vi "Camera setup.vi"() -> ()   [LabVIEW 2012]
uses:
  <vilib>/userDefined/High Color/IMAQdx.ctl
  <vilib>/vision/Calibration.llb/Calibration Reference Points.ctl
  <vilib>/vision/driver/NI_Vision_Acquisition_Software.lvlib
  <vilib>/vision/NI_Vision_Development_Module.lvlib
panel:
  out "ROI":T1
  in  "Attributes":string="[NIIMAQ_HEADER]\nType = 2\nVersion = 8\n\n[CAMERA_DATA]\nAcquisitionAttributes::Bayer::GainB = \"1\"\nAcquisitionAttributes::Bayer::GainG = \"1\"\nAcquisitionAttributes::Bayer::GainR = \"1\"\nAcquisitionAttributes::Bayer::Pattern = \"Use hardware value\"\nAcquisitionAttributes::BitsPerPixel = \"Use hardware value\"\nAcquisitionAttributes::IgnoreFirstFrame = \"false\"\nAcquisitionAttributes::OverwriteMode = \"Get Newest\"\nAcquisitionAttributes::PixelSignedness = \"Signed\"\nAcquisitionAttributes::ReceiveTimestampMode = \"None\"\nAcquisitionAttributes::ShiftPixelBits = \"false\"\nAcquisitionAttributes::SwapPixelBytes = \"false\"\nAcquisitionAttributes::Timeout = \"5000\"\nAcquisitionAttributes::VerticalMirror = \"false\"\nAcquisitionAttributes::VideoMode = \"960x720 RGB24 15.00fps\"\nCameraAttributes::BacklightCompensation::Mode = \"Manual\"\nCameraAttributes::BacklightCompensation::Value = \"false\"\nCameraAttributes::Brightness::Mode = \"Manual\"\nCameraAttributes::Brightness::Value = \"128\"\nCameraAttributes::Contrast::Mode = \"Manual\"\nCameraAttributes::Contrast::Value = \"0.27000000000000002\"\nCameraAttributes::Exposure::Mode = \"Manual\"\nCameraAttributes::Exposure::Value = \"0.015625\"\nCameraAttributes::Gain::Mode = \"Manual\"\nCameraAttributes::Gain::Value = \"254\"\nCameraAttributes::Saturation::Mode = \"Manual\"\nCameraAttributes::Saturation::Value = \"28\"\nCameraAttributes::Sharpness::Mode = \"Manual\"\nCameraAttributes::Sharpness::Value = \"180\"\nCameraAttributes::WhiteBalance::Mode = \"Manual\"\nCameraAttributes::WhiteBalance::Value = \"6299\"\n"
  out "Tank":dbl(slide) scale=0.0..300.0
  in  "Stop Acquisition":bool
  in  "millisecond multiple":u32
  in  "Continuous Acquire image":bool
  out "min index":i32
  out "Gray":T2(plugin-control)
  in  "Smooth Length":i32=5
  out "max index":i32
  out "ROI Out":T2(plugin-control)
  in  "Floc Interface":bool
  out "Reference Points":T3
  in  "Grid Size":cluster{"Max X":u32, "Max Y":u32}
  in  "Grid Descriptor":cluster{"X Step":sgl, "Y Step":sgl, "Unit":T4}={"X Step"=1.0, "Y Step"=1.0, "Unit"=enum."Inch"}
  in  "Calibrate scale":bool
  in  "Folder Path to Store Images":path
  in  "Acquire image":bool
  in  "stop":bool
  out "error out":errorcluster
  out "Image Out":T2(plugin-control)
  in  "Select Camera":T5
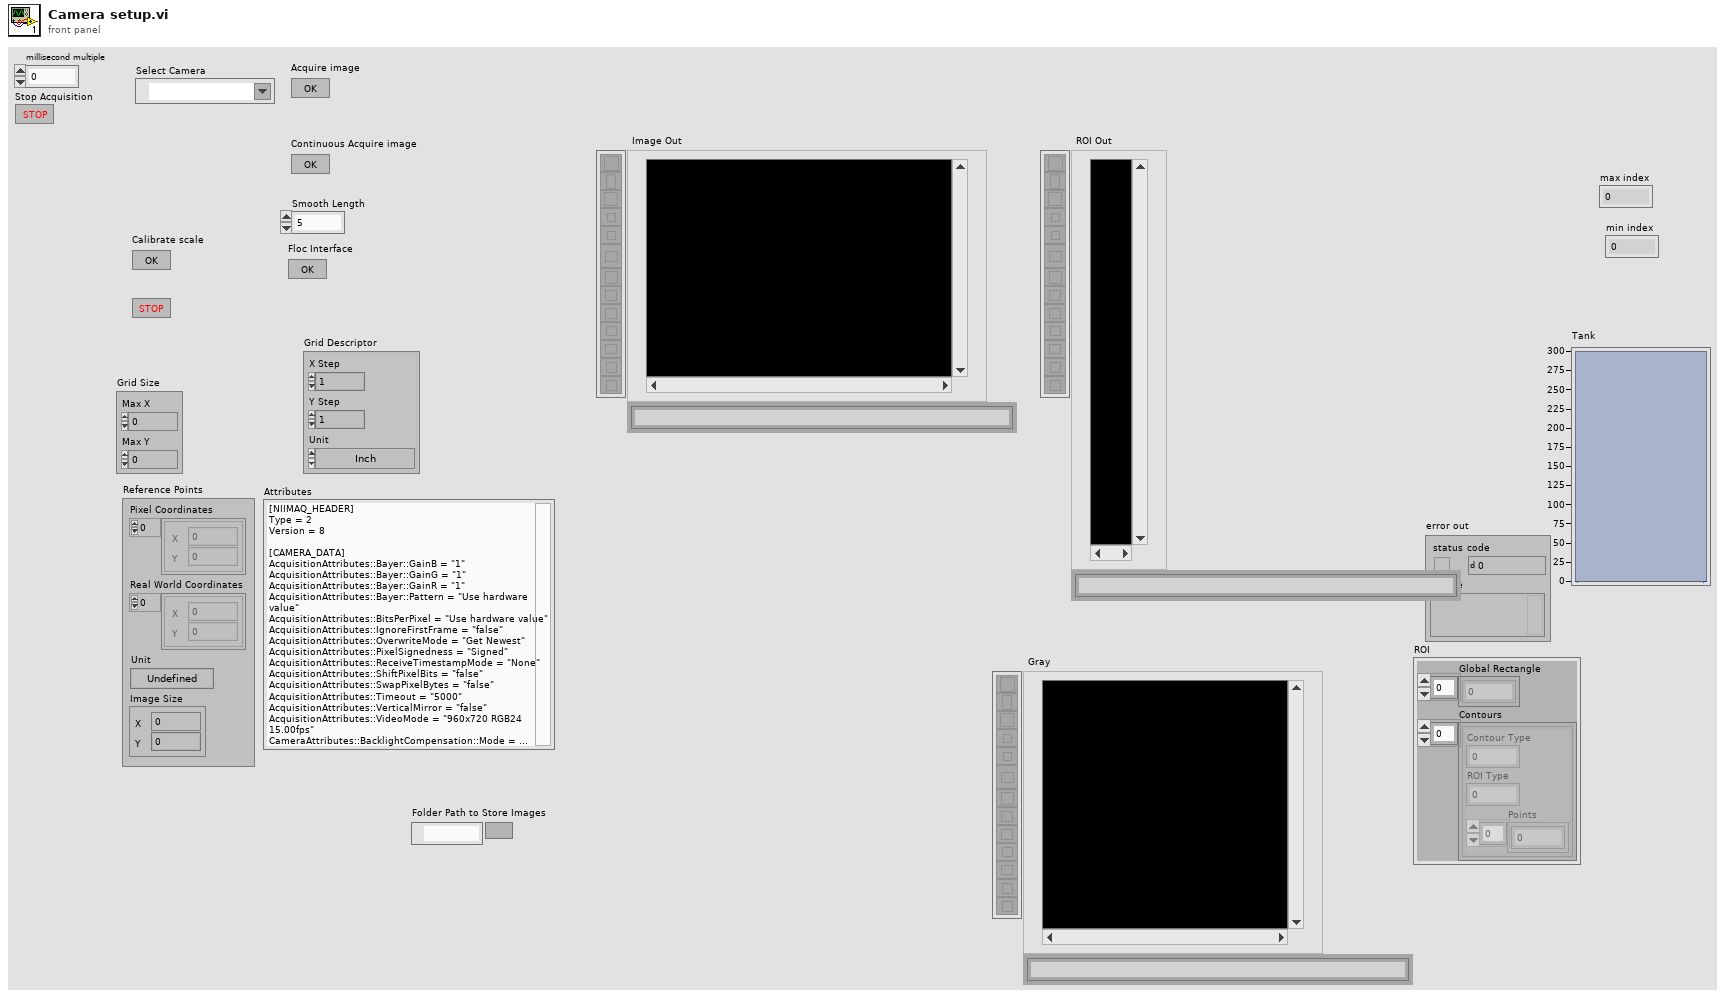
[diagram p1: front panel]
types:
  T1 = cluster{"Global Rectangle":i32[], "Contours":cluster{"Contour Type":u32, "ROI Type":u32, "Points":i32[]}[]}
  T2 = typedef "IMAQ Image.ctl" = refnum<image>
  T3 = typedef "Calibration Reference Points.ctl" = cluster{"Pixel Coordinates":cluster{"X":dbl, "Y":dbl}[], "Real World Coordinates":cluster{"X":dbl, "Y":dbl}[], "Unit":T4, "Image Size":cluster{"X":u32, "Y":u32}}
  T4 = typedef "Image Unit" = enum32{"Undefined", "Angström", "Micrometer", "Millimeter", "Centimeter", "Meter", "Kilometer", "Microinch", "Inch", "Feet", "Nautical miles", "Standard miles", "Steps"}
  T5 = typedef "IMAQdx.ctl" = refnum<k21>
  T6 = typedef "Image Type" = u32
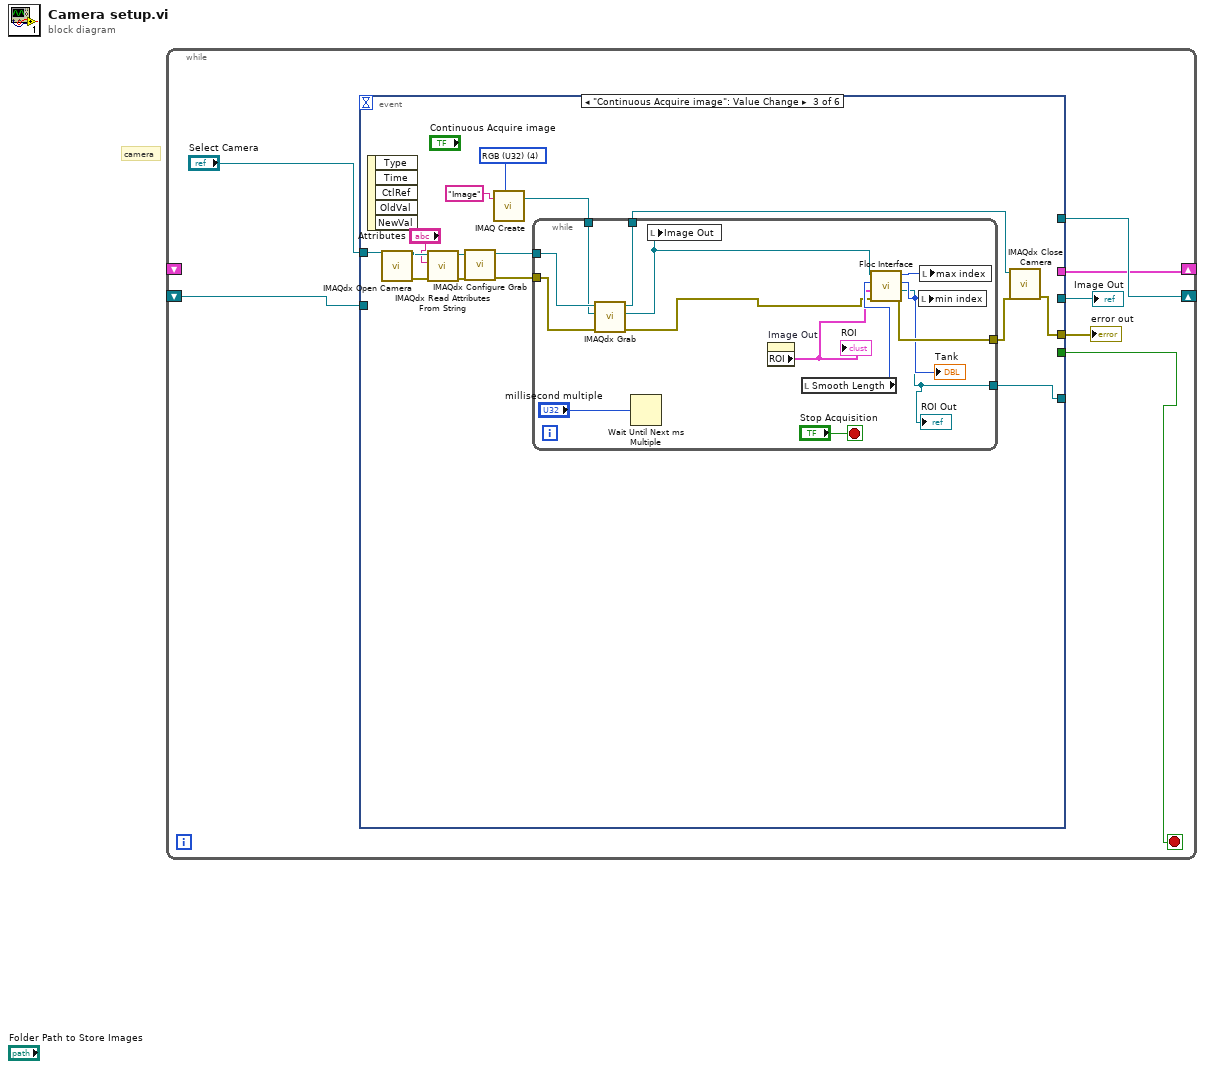
[diagram p0: block diagram]
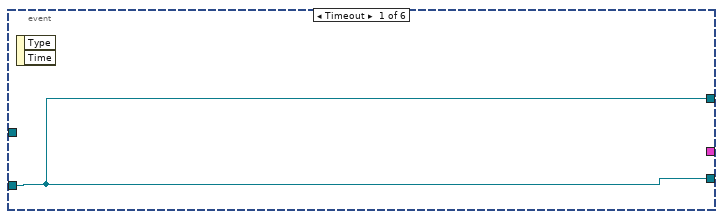
[diagram p2: hidden frame]
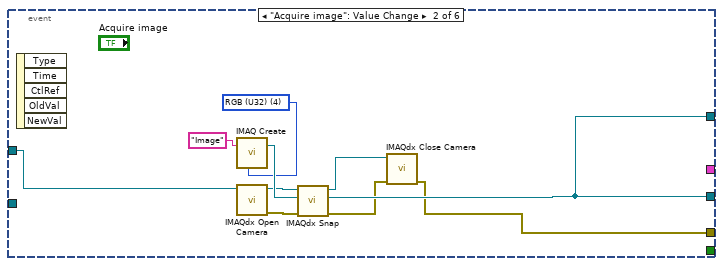
[diagram p3: hidden frame]
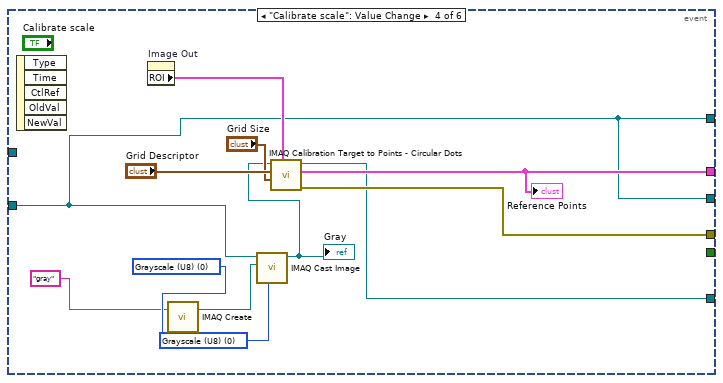
[diagram p4: hidden frame]
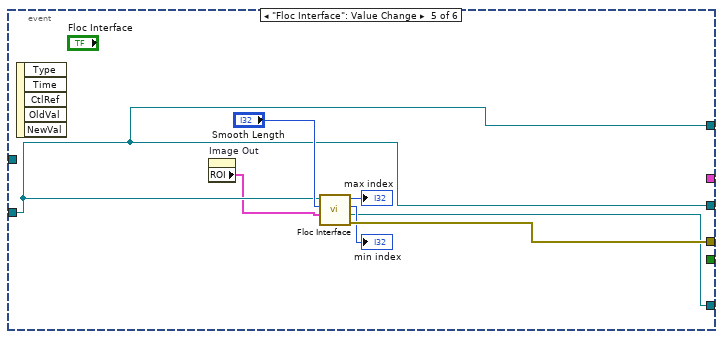
[diagram p5: hidden frame]
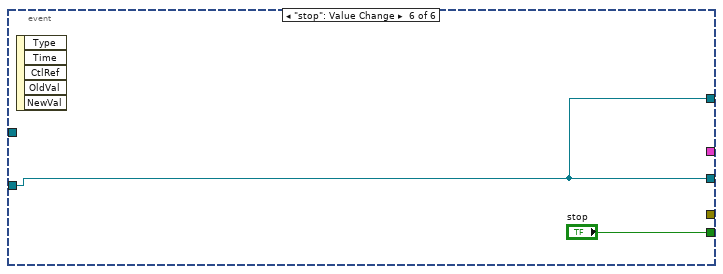
[diagram p6: hidden frame]
diagram:
  # "camera"
  n1 = while {
    shift-right: [w4] -> _
    shift-left: _ -> [w6]
    shift-right: [w3] -> _
    shift-left: _ -> [_]
    stop <- w7 stop-if-true
    n2 = event shown="[2] \"Continuous Acquire image\": Value Change" {
      selector: _ -> [_ _ _ _ _ _]
      dyn-events: _ -> [_ _ _ _ _ _]
      timeout: _ -> [_ _ _ _ _ _]
      tunnel: [_ _ _ _ _ "stop"] -> w7
      tunnel: [w8 w13 _ w48 w61 w67] -> w5
      tunnel: w6 -> [w8 _ _ w48 w61 w67]
      tunnel: [w8 w13 _ w48 w61 w67] -> w4
      tunnel: [_ _ _ w50 _ _] -> w3
      tunnel: [_ w10 w21 w56 w64 _] -> w2
      tunnel: [_ _ w19 w49 w62 _] -> _
      tunnel: "Select Camera" -> [_ w9 w33 _ _ _]
      event Timeout {
        n3 = event-data() -> ()  [unwired: 1 in, 2 out]
      }
      event "Acquire image": Value Change {
        w14 = T6 4 items=["Grayscale (U8)", "Grayscale (I16)", "Grayscale (SGL)", "Complex (CSG)", "RGB (U32)", "HSL (U32)", "RGB (U64)", "Grayscale (U16)"] ("Image Type")
        n4 = event-data() -> ()  [unwired: 1 in, 5 out]
        n5 = call "IMAQ Create"("Image Name"="Image", "Image Type"=w14) -> ("New Image"=w17:T2)  [unwired: 2 in, 2 out]
        n6 = call <vilib>:"IMAQdx Open Camera.vi"("Session In"=w9) -> ("error out"=w16:errorcluster, "Session Out"=w15:T5)  [unwired: 9 in]
        n7 = call <vilib>:"IMAQdx Snap.vi"("error in"=w16, "Image In"=w17, "Session In"=w15) -> ("error out"=w11:errorcluster, "Image Out"=w13:T2, "Session Out"=w12:T5)  [unwired: 6 in]
        n8 = call <vilib>:"IMAQdx Close Camera.vi"("error in"=w11, "Session In"=w12) -> ("error out"=w10:errorcluster)  [unwired: 9 in]
      }
      event "Continuous Acquire image": Value Change {
        w25 = T6 4 items=["Grayscale (U8)", "Grayscale (I16)", "Grayscale (SGL)", "Complex (CSG)", "RGB (U32)", "HSL (U32)", "RGB (U64)", "Grayscale (U16)"] ("Image Type")
        n9 = event-data() -> ()  [unwired: 1 in, 5 out]
        n10 = call <vilib>:"IMAQdx Open Camera.vi"("Session In"=w33) -> ("error out"=w32:errorcluster, "Session Out"=w31:T5)  [unwired: 9 in]
        n11 = call <vilib>:"IMAQdx Read Attributes From String.vi"("error in"=w32, "Attributes String In"="Attributes", "Session In"=w31) -> ("error out"=w29:errorcluster, "Session Out"=w28:T5)  [unwired: 7 out]
        n12 = call <vilib>:"IMAQdx Configure Grab.vi"("error in"=w29, "Session In"=w28) -> ("error out"=w27:errorcluster, "Session Out"=w26:T5)  [unwired: 8 in]
        n13 = call "IMAQ Create"("Image Name"="Image", "Image Type"=w25) -> ("New Image"=w23:T2)  [unwired: 2 in, 2 out]
        n14 = while {
          tunnel: w27 -> [w43]
          tunnel: w26 -> [w42]
          tunnel: w23 -> [w41]
          tunnel: [w40] -> w22
          tunnel: [w39] -> w20
          tunnel: [w34] -> w19
          stop <- "Stop Acquisition" stop-if-true
          n15 = call <vilib>:"IMAQdx Grab.vi"("error in"=w43, "Image In"=w41, "Session In"=w42) -> ("error out"=w35:errorcluster, "Image Out"=w36:T2, "Session Out"=w40:T5)  [unwired: 5 in, 1 out]
          n16 = Wait Until Next ms Multiple(millisecond multiple="millisecond multiple") -> ()  [unwired: 1 out]
          n17 = local write "Image Out"(w36) -> ()
          n18 = property on="Image Out" class="ImageControl"() -> ("ROI"=w37:T1)  [unwired: 2 in, 2 out]
          "ROI" <- w37
          n19 = local read "Smooth Length"() -> (w45:i32)
          n20 = call "Floc Interface.vi"("error in"=w35, "ROI"=w37, "Smooth Length"=w45, "Image"=w36) -> ("error out"=w39:errorcluster, "ROI Out"=w34:T2, "min index"=w38:i32, "max index"=w44:i32)  [unwired: 2 in, 2 out]
          "Tank" <- w38
          "ROI Out" <- w34
          n21 = local write "min index"(w38) -> ()
          n22 = local write "max index"(w44) -> ()
        }
        n23 = call <vilib>:"IMAQdx Close Camera.vi"("error in"=w20, "Session In"=w22) -> ("error out"=w21:errorcluster)  [unwired: 9 in]
      }
      event "Calibrate scale": Value Change {
        w52 = T6 0 items=["Grayscale (U8)", "Grayscale (I16)", "Grayscale (SGL)", "Complex (CSG)", "RGB (U32)", "HSL (U32)", "RGB (U64)", "Grayscale (U16)"] ("Image Type")
        w55 = T6 0 items=["Grayscale (U8)", "Grayscale (I16)", "Grayscale (SGL)", "Complex (CSG)", "RGB (U32)", "HSL (U32)", "RGB (U64)", "Grayscale (U16)"] ("Image Type")
        n24 = event-data() -> ()  [unwired: 1 in, 5 out]
        n25 = property on="Image Out" class="ImageControl"() -> ("ROI"=w57:T1)  [unwired: 2 in, 2 out]
        n26 = call "IMAQ Create"("Image Name"="gray", "Image Type"=w55) -> ("New Image"=w53:T2)  [unwired: 2 in, 2 out]
        n27 = call "IMAQ Cast Image"("Image Type"=w52, "Image Dst"=w53, "Image Src"=w48) -> ("Image Dst Out"=w51:T2)  [unwired: 7 in, 1 out]
        "Gray" <- w51
        n28 = call "IMAQ Calibration Target to Points - Circular Dots"("ROI Descriptor"=w57, "Grid Size"="Grid Size", "Grid Descriptor"="Grid Descriptor", "Target Image"=w51) -> ("error out"=w56:errorcluster, "Reference Points"=w50:T3, "Target Image (dup)"=w49:T2)  [unwired: 5 in]
        "Reference Points" <- w50
      }
      event "Floc Interface": Value Change {
        n29 = event-data() -> ()  [unwired: 1 in, 5 out]
        n30 = property on="Image Out" class="ImageControl"() -> ("ROI"=w60:T1)  [unwired: 2 in, 2 out]
        n31 = call "Floc Interface.vi"("ROI"=w60, "Smooth Length"="Smooth Length", "Image"=w61) -> ("error out"=w64:errorcluster, "ROI Out"=w62:T2, "min index"=→"min index":i32, "max index"=→"max index":i32)  [unwired: 3 in, 2 out]
      }
      event "stop": Value Change {
        n32 = event-data() -> ()  [unwired: 1 in, 5 out]
      }
    }
    "Image Out" <- w5
    "error out" <- w2
  }
